vi "arrays manipulations.vi"() -> ()   [LabVIEW 2020]
panel:
  out "output array":dbl[](array[numeric])
  out "appended array":dbl[](array[numeric])
  out "secondarray":dbl[](array[numeric])
  out "firstarray":dbl[](array[numeric])
  out "subarray":dbl[][](array[numeric])
  out "Array":dbl[][](array[numeric])
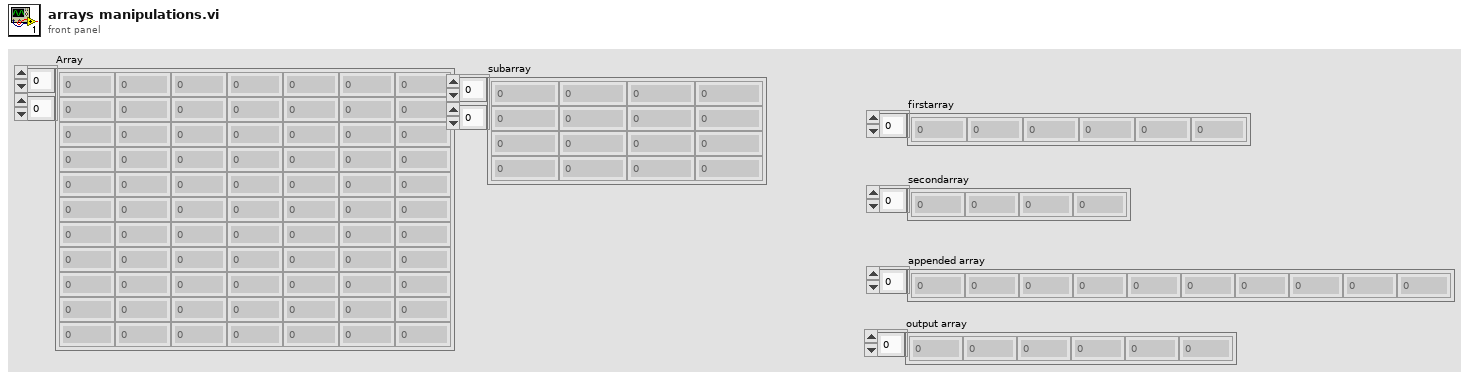
[diagram p1: front panel]
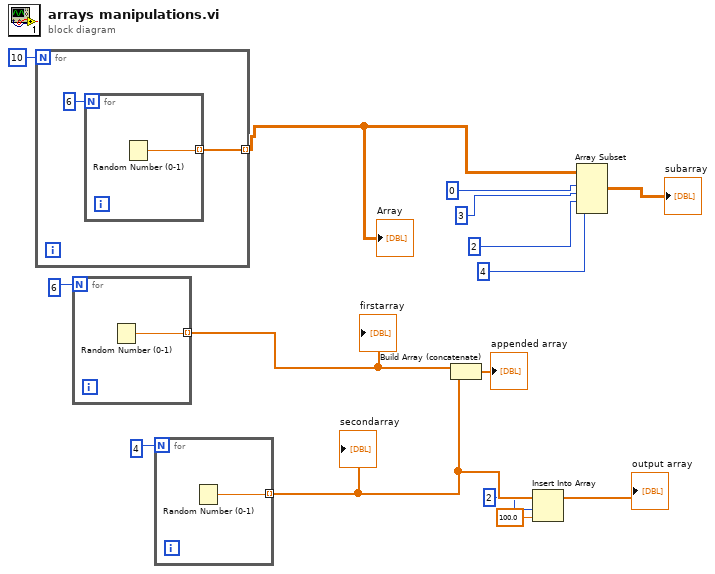
[diagram p0: block diagram]
diagram:
  n1 = for {
    N: 10 -> [_]
    tunnel: [w16] -> w10 mode=indexing
    n2 = for {
      N: 6 -> [_]
      tunnel: [w18] -> w16 mode=indexing
      n3 = Random Number (0-1)() -> (number: 0 to 1=w18:dbl)
    }
  }
  "Array" <- w10
  n4 = for {
    N: 6 -> [_]
    tunnel: [w19] -> w7 mode=indexing
    n5 = Random Number (0-1)() -> (number: 0 to 1=w19:dbl)
  }
  "firstarray" <- w7
  n6 = for {
    N: 4 -> [_]
    tunnel: [w20] -> w4 mode=indexing
    n7 = Random Number (0-1)() -> (number: 0 to 1=w20:dbl)
  }
  "secondarray" <- w4
  n8 = Build Array (concatenate)(w7, w4) -> (→"appended array":dbl[])
  n9 = Insert Into Array(array=w4, index=2, new element=100.0 ("new element/subarray")) -> (→"output array":dbl[])
  n10 = Array Subset(array=w10, index (row)=0, length (row)=3, index (col)=2, length (col)=4) -> (→"subarray":dbl[][])
